vi "disconnect From All Cyclones.vi"(8 "error in":errorcluster) -> (0 "error out":errorcluster)   [LabVIEW 2021, in "CycloneControlSDK.lvlib"]
doc: "extern \"C\" void _cdecl disconnectFromAllCyclones(void);"
uses:
  CycloneControlSDK.lvlib
  CycloneControlSDK_64.dll
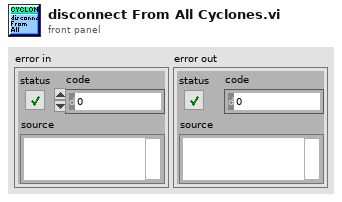
[diagram p1: front panel]
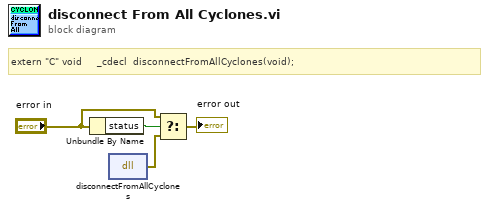
[diagram p0: block diagram]
diagram:
  # "extern \"C\" void     _cdecl  disconnectFromAllCyclones(void);"
  n1 = Unbundle By Name("error in") -> ("status"=w4:bool)
  n2 = dll-call lib="C:/PEMicro/cyclone/cycloneControl/controlsdk/examples/labview2018/user.lib/CycloneControlSDK/CycloneControlSDK_64.dll" fn="disconnectFromAllCyclones"() -> (error out=w1:errorcluster)  [unwired: 4 in, 1 out]
  n3 = Select(t="error in", s=w4, f=w1) -> (s? t:f=→"error out":errorcluster)
